vi "XORFilter.vi"(0 "Image Src 1":T1, 1 "Filtered Image Dst 1":T1, 2 "Processed Image Dst 2":T1, 3 "Image Src 2":T1, 4 "Filtered Image Dst 2":T1, 5 "Processed Image Dst 2":T1, 7 "XOR Image Dst":T1, 9 "Threshold Range":cluster{"Lower value":sgl, "Upper value":sgl}={"Lower value"=240.0, "Upper value"=255.0} {"Upper value" format="%.2f"; "Lower value" format="%.2f"}) -> (14 "XOR Image Dst Out":T1, 15 "Image Dst 1 Out":T1, 16 "Image Dst 2 Out":T1)   [LabVIEW 2011]
uses:
  <vilib>/vision/Image Controls.llb/IMAQ Image.ctl
  <vilib>/vision/NI_Vision_Development_Module.lvlib
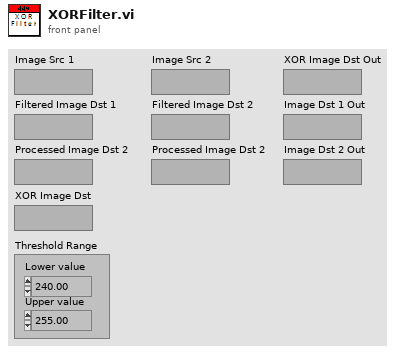
[diagram p1: front panel]
types:
  T1 = typedef "IMAQ Image.ctl" = refnum<image>
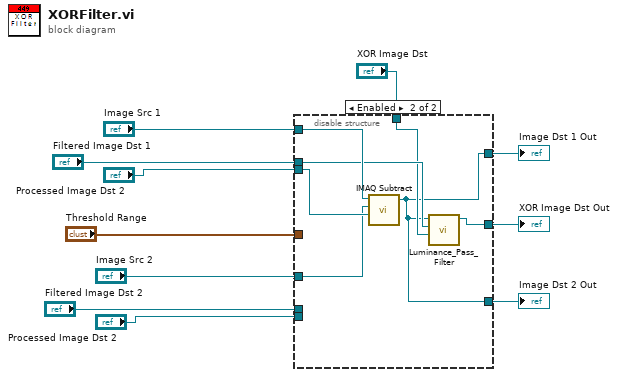
[diagram p0: block diagram]
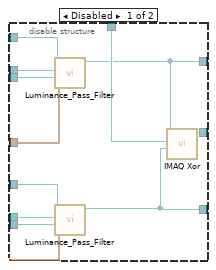
[diagram p2: hidden frame]
diagram:
  n1 = disable-structure shown="Enabled" {
    disable-tunnel: "Image Src 1" -> [w22 w29]
    disable-tunnel: "Filtered Image Dst 1" -> [w21 w26]
    disable-tunnel: "Processed Image Dst 2" -> [w20 w28]
    disable-tunnel: "Image Src 2" -> [w19 w27]
    disable-tunnel: "Filtered Image Dst 2" -> [w18 _]
    disable-tunnel: "Processed Image Dst 2" -> [w17 _]
    disable-tunnel: "XOR Image Dst" -> [w16 w25]
    disable-tunnel: [w15 w24] -> w4
    disable-tunnel: [w14 w23] -> w3
    disable-tunnel: [w13 w23] -> w2
    disable-tunnel: "Threshold Range" -> [w12 _]
    frame Disabled {
      n2 = call "Luminance_Pass_Filter.vi"("Threshold Range"=w12, "Processed Image Dst"=w20, "Filtered Image Dst"=w21, "Image Src"=w22) -> ("Image Dst Out"=w13:T1)  [unwired: 7 in]
      n3 = call "Luminance_Pass_Filter.vi"("Threshold Range"=w12, "Processed Image Dst"=w17, "Filtered Image Dst"=w18, "Image Src"=w19) -> ("Image Dst Out"=w14:T1)  [unwired: 7 in]
      n4 = call "IMAQ Xor"("Image Src B"=w14, "Image Dst"=w16, "Image Src A"=w13) -> ("Image Dst Out"=w15:T1)  [unwired: 7 in, 1 out]
    }
    frame Enabled {
      n5 = call "IMAQ Subtract"("Image Src A"=w29, "Image Dst"=w27, "Image Src B"=w28) -> ("Image Dst Out"=w23:T1)  [unwired: 4 in, 1 out]
      n6 = call "Luminance_Pass_Filter.vi"("Processed Image Dst"=w25, "Filtered Image Dst"=w26, "Image Src"=w23) -> ("Image Dst Out"=w24:T1)  [unwired: 8 in]
    }
  }
  "XOR Image Dst Out" <- w4
  "Image Dst 1 Out" <- w2
  "Image Dst 2 Out" <- w3
